vi "Send ADC.vi"(8 "error in (no error)":errorcluster, 9 "Channel":enum16{"2", "1"}(ring), 10 "VISA resource name":refnum<visa-resource-name>, 11 "Serial Device in":refnum<class "Serial Device.lvclass">) -> (0 "error out":errorcluster, 1 "Response":i32, 2 "VISA resource name 2":refnum<visa-resource-name>, 3 "Serial Device out":refnum<class "Serial Device.lvclass">, 4 "command":string)   [LabVIEW 2020, in "Serial Device.lvclass"]
uses:
  Serial Device.lvclass
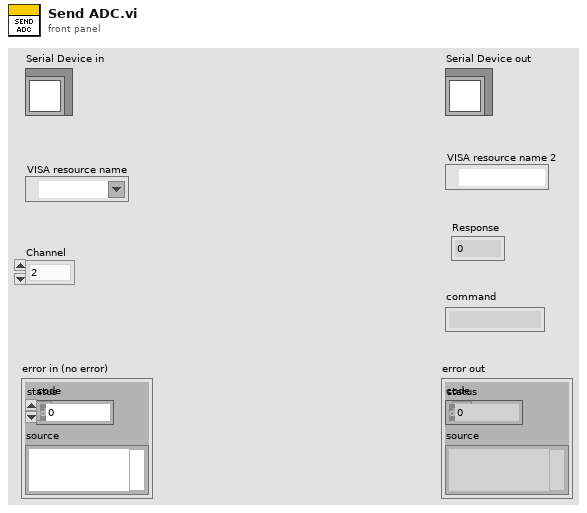
[diagram p1: front panel]
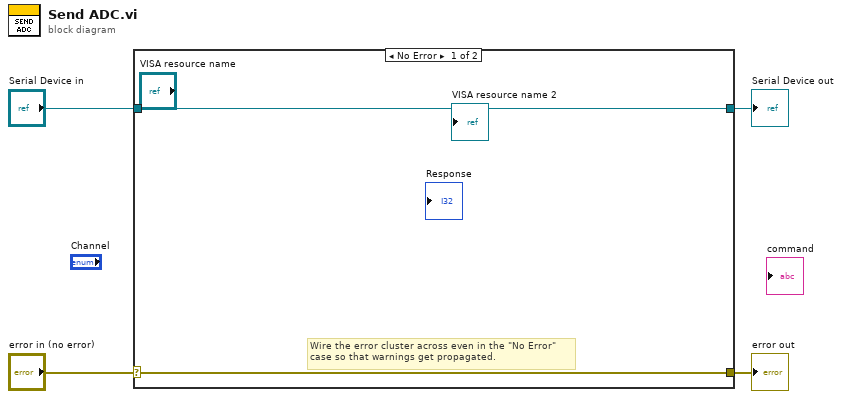
[diagram p0: block diagram]
diagram:
  n1 = case shown="No Error" "error in (no error)" {
    selector: "error in (no error)" -> [w5 w8]
    tunnel: [w5 w8] -> w3
    tunnel: [w6 w7] -> w1
    tunnel: "Serial Device in" -> [w6 w7]
    frame No Error {
      # "Wire the error cluster across even in the \"No Error\"\ncase so that warnings get propagated."
    }
    frame Error {
    }
  }
  "error out" <- w3
  "Serial Device out" <- w1
